vi "Save Settings to XML.vi"() -> ()   [LabVIEW 2015, in "Settings.lvlib"]
uses:
  Settings.lvlib
  Settings.ctl
  Camera/Camera Configuration.ctl
  Logging/Logging Configuration.ctl
  XYZStage/XYZStage Configuration.ctl
  DM/DM Configuration.ctl
  Automation/Automation Configuration.ctl
  V7001/V7001 Configuration.ctl
  AOD/AOD Configuration.ctl
  <vilib>/Utility/xml.llb/Write to XML File(string).vi
  Camera/Camera.lvlib
  Logging/Logging.lvlib
  AOD/AOD.lvlib
  V7001/V7001.lvlib
  Automation/Automation.lvlib
  DM/DM.lvlib
  XYZStage/XYZStage.lvlib
panel:
  in  "error in (no error)":errorcluster
  out "error out":errorcluster
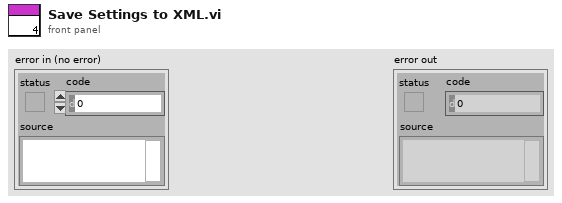
[diagram p1: front panel]
types:
  T1 = typedef "Settings.lvlib/Settings.ctl" = cluster{"Camera Configuration":T2, "Logging Configuration":T3, "XYZ Configuration":T4, "DM Configuration":T5, "Automation Configuration":T6, "V7001 Configuration":T7, "AOD Configuration":T8}
  T2 = typedef "Camera.lvlib/Camera Configuration.ctl" = cluster{"Camera Index":u32}
  T3 = typedef "Logging.lvlib/Logging Configuration.ctl" = cluster{"Log File Base Path":path}
  T4 = typedef "XYZStage.lvlib/XYZStage Configuration.ctl" = cluster{"VISA resource name":refnum<visa-resource-name>, "Timeout (3sec)":u32}
  T5 = typedef "DM.lvlib/DM Configuration.ctl" = cluster{"Selected Profile":string, "dm out":cluster{"type":i32, "ID":i32, "size":i32, "@dummy control@":i8, "@dummy control@":i8, "@dummy control@":i8, "@dummy control@":i8, "lutName":u64}}
  T6 = typedef "Automation.lvlib/Automation Configuration.ctl" = cluster{" Index":u32}
  T7 = typedef "V7001.lvlib/V7001 Configuration.ctl" = cluster{" Index":u32}
  T8 = typedef "AOD.lvlib/AOD Configuration.ctl" = cluster{"Physical Channel":tag, "Maximum Value":dbl, "Minimum Value":dbl, "Update Rate":dbl}
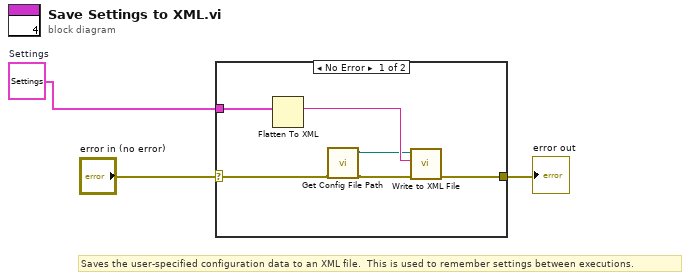
[diagram p0: block diagram]
diagram:
  w1 = T1 {"Camera Configuration"={"Camera Index"=0}, "Logging Configuration"={"Log File Base Path"=path ""}, "XYZ Configuration"={"VISA resource name"="", "Timeout (3sec)"=0}, "DM Configuration"={"Selected Profile"="", "dm out"={"type"=0, "ID"=0, "size"=0, "@dummy control@"=0, "@dummy control@"=0, "@dummy control@"=0, "@dummy control@"=0, "lutName"=0}}, "Automation Configuration"={" Index"=0}, "V7001 Configuration"={" Index"=0}, "AOD Configuration"={"Physical Channel"="Dev1/ao0:1", "Maximum Value"=0.0, "Minimum Value"=1.0, "Update Rate"=192000.0}}  # Settings
  # "Saves the user-specified configuration data to an XML file.  This is used to remember settings between executions."
  n1 = case shown="No Error" "error in (no error)" {
    selector: "error in (no error)" -> [w4 w10]
    tunnel: [w7 w10] -> w2
    tunnel: w1 -> [w9 _]
    frame No Error {
      n2 = Flatten To XML(anything=w9) -> (xml string=w8:string)
      n3 = call "Get Config File Path.vi"("error in (no error)"=w4) -> ("error out"=w5:errorcluster, "XML File Path"=w6:path)  [unwired: 9 in]
      n4 = call-poly <vilib>:"Write to XML File.vi"("error in (no error)"=w5, "XML Input"=w8, "XML File Path"=w6) -> ("error out"=w7:errorcluster)  [unwired: 6 in, 2 out]
    }
    frame Error {
    }
  }
  "error out" <- w2
